vi "PXI-Enumerate Channels.vi"(0 "Devices":T1[](array[typedef]), 11 "error in (no error)":errorcluster) -> (4 "Channels By Device":cluster{"Out":string[], "In":string[]}[](array[cluster]), 8 "Channels (1D)":cluster{"Out":string[], "In":string[]}, 15 "error out":errorcluster)   [LabVIEW 2020]
uses:
  Type Defs/PXI-Device Spec.ctl
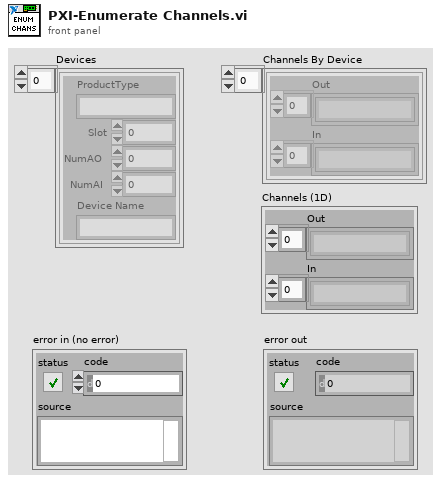
[diagram p1: front panel]
types:
  T1 = typedef "PXI-Device Spec.ctl" = cluster{"Slot":i32, "ProductType":string, "NumAO":i32, "NumAI":i32, "Device Name":string}
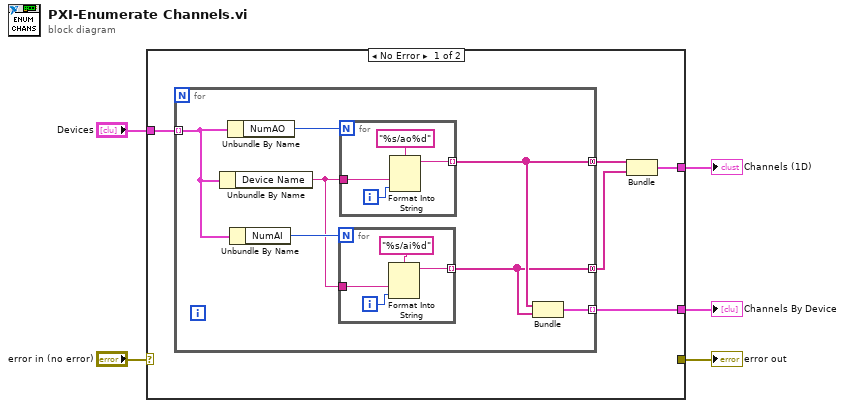
[diagram p0: block diagram]
diagram:
  n1 = case shown="No Error" "error in (no error)" {
    selector: "error in (no error)" -> [_ w26]
    tunnel: "Devices" -> [w10 _]
    tunnel: [w9 _] -> w4
    tunnel: [w6 _] -> w3
    tunnel: [_ w26] -> w1
    frame No Error {
      n2 = for {
        tunnel: w10 -> [w15] mode=indexing
        tunnel: [w13] -> w8 mode=concatenating
        tunnel: [w12] -> w7 mode=concatenating
        tunnel: [w11] -> w9 mode=indexing
        n3 = Unbundle By Name(w15) -> ("Device Name"=w14:string)
        n4 = Unbundle By Name(w15) -> ("NumAO"=w17:i32)
        n5 = Unbundle By Name(w15) -> ("NumAI"=w16:i32)
        n6 = for {
          N: w16 -> [_]
          tunnel: w14 -> [w20]
          tunnel: [w18] -> w12 mode=indexing
          i -> [w19]
          n7 = Format Into String(format string="%s/ai%d", w20, w19) -> (resulting string=w18:string)  [unwired: 2 in, 1 out]
        }
        n8 = for {
          N: w17 -> [_]
          tunnel: w14 -> [w24]
          tunnel: [w22] -> w13 mode=indexing
          i -> [w23]
          n9 = Format Into String(format string="%s/ao%d", w24, w23) -> (resulting string=w22:string)  [unwired: 2 in, 1 out]
        }
        n10 = Bundle(w13, w12) -> (w11:cluster{string[], string[]})  [unwired: 1 in]
      }
      n11 = Bundle(w8, w7) -> (w6:cluster{string[], string[]})  [unwired: 1 in]
    }
    frame Error {
    }
  }
  "error out" <- w1
  "Channels By Device" <- w4
  "Channels (1D)" <- w3
